vi "SAM-Modulation Level Correction.vi"(0 "SAM":T1, 11 "error in (no error)":errorcluster) -> (8 "Correction (dB)":dbl, 15 "error out":errorcluster)   [LabVIEW 2020]
uses:
  SAM Params.ctl
  Utility VIs/Math VIs/Linear to dB (scalar).vi
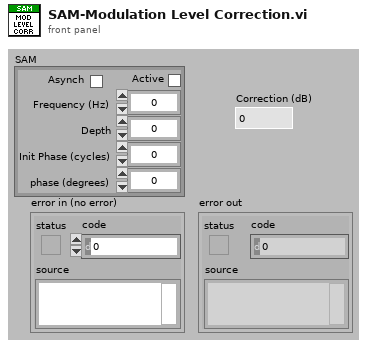
[diagram p1: front panel]
types:
  T1 = typedef "SAM Params.ctl" = cluster{"Active":bool, "Frequency (Hz)":dbl, "Depth":dbl, "Init Phase (cycles)":dbl, "phase (degrees)":dbl, "Asynch":bool}
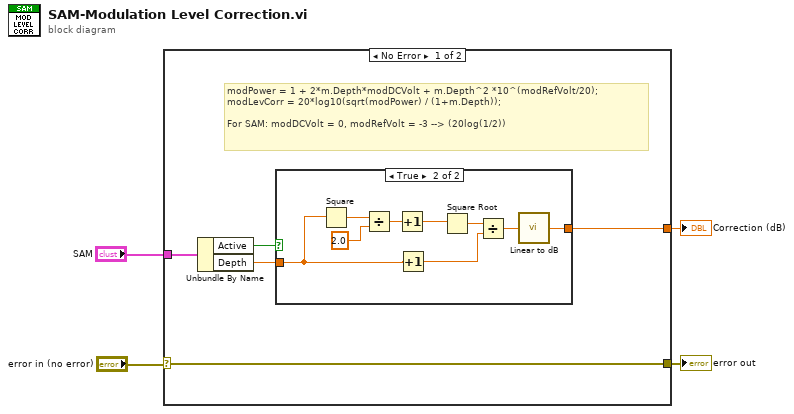
[diagram p0: block diagram]
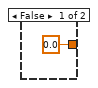
[diagram p2: hidden frame]
diagram:
  n1 = case shown="No Error" "error in (no error)" {
    selector: "error in (no error)" -> [w9 w20]
    tunnel: [w9 w20] -> w3
    tunnel: "SAM" -> [w8 _]
    tunnel: [w5 _] -> w1
    frame No Error {
      # "modPower = 1 + 2*m.Depth*modDCVolt + m.Depth^2 *10^(modRefVolt/20);\nmodLevCorr = 20*log10(sqrt(modPower) / (1+m.Depth));\n\nFor SAM: modDCVolt = 0, modRefVolt = -3 --> (20log(1/2))"
      n2 = Unbundle By Name(w8) -> ("Active"=w6:bool, "Depth"=w7:dbl)
      n3 = case shown="True" w6 {
        tunnel: w7 -> [_ w15]
        tunnel: [0.0 ("dB") w11] -> w5
        frame False {
        }
        frame True {
          n4 = Square(x=w15) -> (x^2=w19:dbl)
          n5 = Divide(x=w19, y=2.0) -> (x/y=w17:dbl)
          n6 = Increment(x=w17) -> (x+1=w16:dbl)
          n7 = Increment(x=w15) -> (x+1=w13:dbl)
          n8 = Square Root(x=w16) -> (sqrt(x)=w14:dbl)
          n9 = Divide(x=w14, y=w13) -> (x/y=w12:dbl)
          n10 = call-poly "Linear to dB.vi"("Linear"=w12) -> ("dB"=w11:dbl)
        }
      }
    }
    frame Error {
    }
  }
  "error out" <- w3
  "Correction (dB)" <- w1
